vi "Detect Bump.vi"(11 "y angle":dbl) -> (3 "Bumpy Terrain":bool)   [LabVIEW 2017]
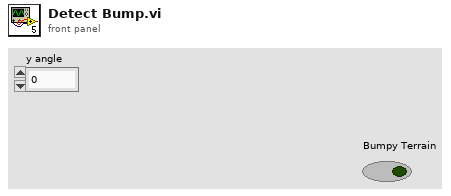
[diagram p1: front panel]
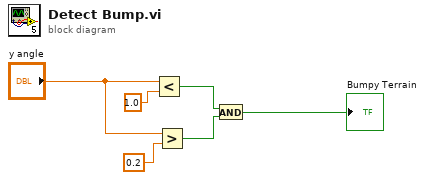
[diagram p0: block diagram]
diagram:
  n1 = Less?(x="y angle", y=1.0) -> (x < y?=w3:bool)
  n2 = Greater?(x="y angle", y=0.2) -> (0:w2:bool)
  n3 = And(x=w3, y=w2) -> (x .and. y?=→"Bumpy Terrain":bool)
